vi "Get Report Type.vi"(0 "report in":refnum<class "NI_Excel.lvclass">, 11 "error in (no error)":errorcluster) -> (4 "report out":refnum<class "NI_Excel.lvclass">, 8 "report type":T1(ring)=enum."HTML", 15 "error out":errorcluster)   [LabVIEW 2020, in "NI_Excel.lvclass"]
doc: "This VI is deprecated. Use the following VI instead:\n\nvi.lib\\Utility\\NIReport.llb\\Report Type.vi\n\nReturns the report type, such as standard, HTML, Word, or Excel, of a specified report."
uses:
  <vilib>/Utility/NIReport.llb/Excel/NI_Excel.lvclass
panel:
  # "This VI is deprecated. Use the following VI instead:\n\nvi.lib\\Utility\\NIReport.llb\\Report Type.vi"
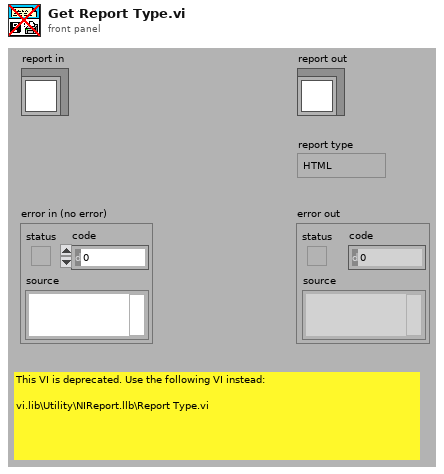
[diagram p1: front panel]
types:
  T1 = enum16{"Standard Report", "HTML", "Word", "Excel"}
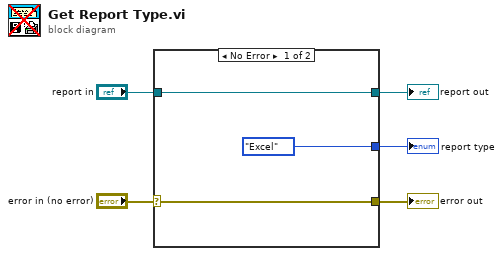
[diagram p0: block diagram]
diagram:
  n1 = case shown="No Error" "error in (no error)" {
    selector: "error in (no error)" -> [w8 w10]
    tunnel: [w8 w10] -> w4
    tunnel: [w7 w9] -> w2
    tunnel: "report in" -> [w7 w9]
    tunnel: [T1."Excel" ("output element") _] -> w1
    frame No Error {
    }
    frame Error {
    }
  }
  "error out" <- w4
  "report out" <- w2
  "report type" <- w1
